vi "external cmd - open and read file.vi"(0 "files array":path[](array[path])) -> (4 "commands":cluster{path, string[], i32[]}, 8 "file has commands":bool)   [LabVIEW 2010]
panel:
  out "line of the command in the file":i32[](array[numeric])
  out "filename":path
  out "list of commands":string[](array[string])
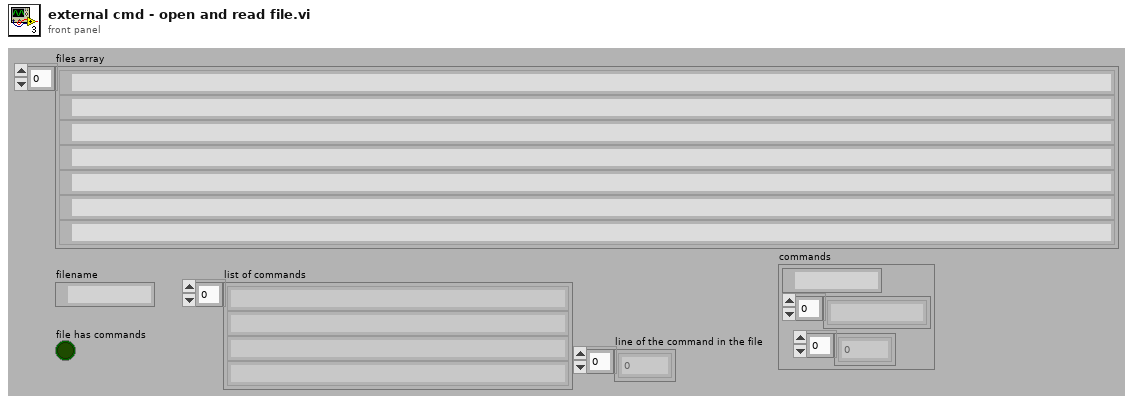
[diagram p1: front panel]
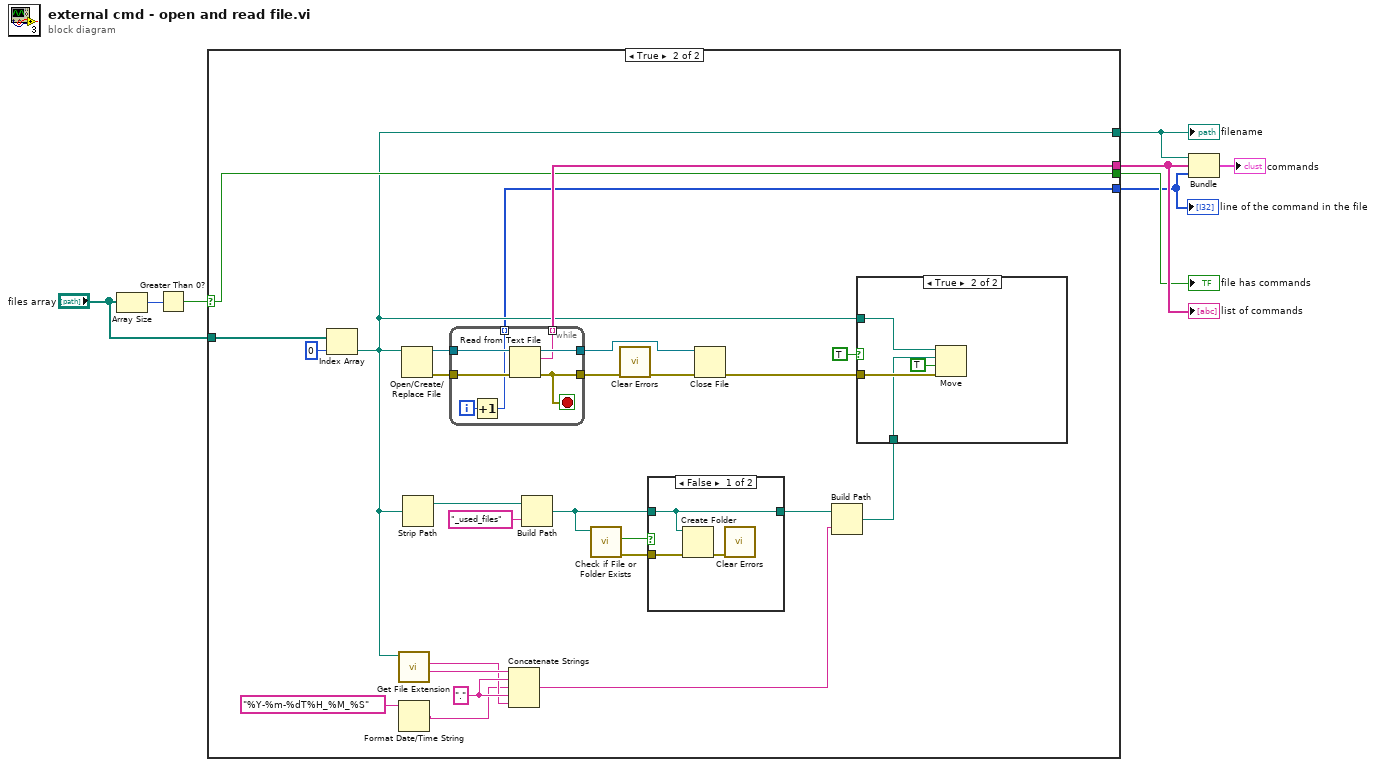
[diagram p0: block diagram]
diagram:
  n1 = Array Size(array="files array") -> (size(s)=w7:i32)
  n2 = Greater Than 0?(x=w7) -> (x > 0?=w8:bool)
  n3 = case shown="True" w8 {
    selector: w8 -> [w9 w12]
    tunnel: "files array" -> [_ w35]
    tunnel: [_ w13] -> w5
    tunnel: [w9 w12] -> w4
    tunnel: [_ w11] -> w3
    tunnel: [_ w10] -> w2
    frame False {
    }
    frame True {
      w21 = "." ("string")
      n4 = Index Array(array=w35, index=0) -> (element=w11:path)
      n5 = call <vilib>:"Get File Extension.vi"("file"=w11) -> ("filename without extension"=w22:string, "lowercase file extension"=w17:string)  [unwired: 7 in, 2 out]
      n6 = Format Date/Time String(time format string (%c)="%Y-%m-%dT%H_%M_%S") -> (date/time string=w15:string)  [unwired: 2 in]
      n7 = Open/Create/Replace File(file path (use dialog)=w11) -> (refnum out=w32:refnum<file>, error out=w33:errorcluster)  [unwired: 5 in, 1 out]
      n8 = Strip Path(path=w11) -> (stripped path=w28:path)  [unwired: 1 out]
      n9 = while {
        tunnel: w33 -> [w42]
        tunnel: w32 -> [w41]
        tunnel: [w39] -> w31
        tunnel: [w40] -> w26
        tunnel: [w38] -> w13 mode=indexing
        tunnel: [w36] -> w10 mode=indexing
        i -> [w37]
        stop <- w39 stop-if-true
        n10 = Increment(x=w37) -> (x+1=w36:i32)
        n11 = Read from Text File(file (use dialog)=w41, error in=w42) -> (refnum out=w40:refnum<file>, text=w38:string, error out=w39:errorcluster)  [unwired: 2 in, 1 out]
      }
      n12 = Concatenate Strings(w22, w21, w15, w21, w17) -> (w19:string)
      n13 = Build Path(base path=w28, name or relative path="_used_files") -> (appended path=w25:path)
      n14 = call <vilib>:"Check if File or Folder Exists.vi"("path"=w25) -> ("error out"=w30:errorcluster, "file or folder exists?"=w29:bool)  [unwired: 8 in, 1 out]
      n15 = call <vilib>:"Clear Errors.vi"("error in (no error)"=w31) -> ("error out"=w24:errorcluster)  [unwired: 6 in]
      n16 = case shown="False" w29 {
        tunnel: w30 -> [w48 _]
        tunnel: w25 -> [w47 w50]
        tunnel: [w47 w50] -> w20
        frame False {
          n17 = Create Folder(path (use dialog)=w47, error in=w48) -> (error out=w49:errorcluster)  [unwired: 1 in, 2 out]
          n18 = call <vilib>:"Clear Errors.vi"("error in (no error)"=w49) -> ()  [unwired: 6 in, 1 out]
        }
        frame True {
        }
      }
      n19 = Close File(refnum=w26, error in=w24) -> (error out=w23:errorcluster)  [unwired: 1 out]
      n20 = Build Path(base path=w20, name or relative path=w19) -> (appended path=w18:path)
      n21 = case shown="True" TRUE {
        tunnel: w23 -> [_ w46]
        tunnel: w11 -> [_ w44]
        tunnel: w18 -> [_ w43]
        frame False {
        }
        frame True {
          n22 = Move(source path=w44, error in=w46, 9:TRUE ("overwrite (F)"), 10:w43) -> ()  [unwired: 1 in, 3 out]
        }
      }
    }
  }
  "list of commands" <- w5
  "filename" <- w3
  "file has commands" <- w4
  "line of the command in the file" <- w2
  n23 = Bundle(w3, w5, w2) -> (→"commands":cluster{path, string[], i32[]})  [unwired: 1 in]
